vi "Emballage_BDD_lecutreCommandeNonTerminé.vi"(8 "entrée d'erreur (pas d'erreur)":errorcluster) -> (0 "sortie d'erreur":errorcluster, 2 "Cmd_nonFini":string[](array[string]), 3 "Liste des champs à lire 2":string[][](array[string]))   [LabVIEW 2020]
uses:
  Modules/FS/60_FS_Controles/60_FS_SetGet.ctl
  <vilib>/addons/database/Connection.llb/DB Tools Open Connec (Path).vi
  <vilib>/addons/database/Connection.llb/Conn Execute.vi
  <vilib>/addons/database/Recordset.llb/Rec Fetch Recordset Data (R).vi
  <vilib>/addons/database/Recordset.llb/Rec Destroy - Connection.vi
  <vilib>/addons/database/NI_Database_API.lvlib
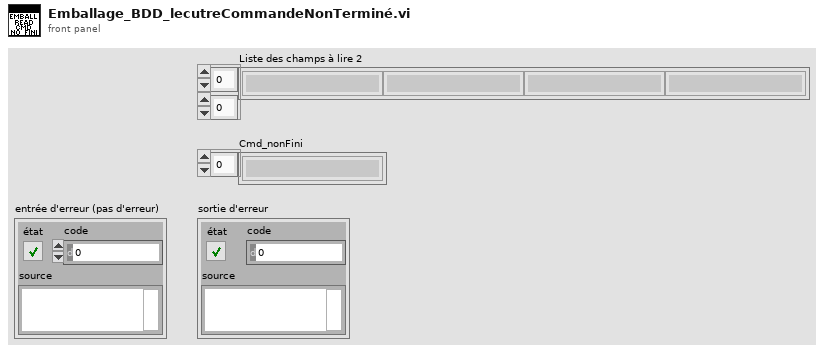
[diagram p1: front panel]
types:
  T1 = typedef "60_FS_SetGet.ctl" = enum16{"set", "get"}
  T2 = typedef "Emballage_BDD_param_Produit.ctl" = cluster{"No_Valve_FAS":string, "suffixe":string, "designation":string, "indice_produit":string, "code_barre_fixe":string, "affiche_code_barre_client":string, "affiche_no_client":string, "Nb_vlve_par_carton":u16, "melange_des_lots_possible":string, "id_article":string, "Indice_Rev":string, "Famille":string, "date":string, "code_barre_fixe_Fin":string, "Longeur_No_Serie":string}
  T3 = typedef "60_FS_CLT_Chemins.ctl" = cluster{"Racine_local":path, "Racine_reseau":path, "Racine_Support_Application":path, "Fichier_Journalisation":path, "Connexion_BDD_VSX":path, "Connexion_BDD_PLZ":path}
  T4 = typedef "NI_Database_API.lvlib/Conn ObjectReference.ctl" = refnum<k1>
  T5 = typedef "NI_Database_API.lvlib/Rec ObjectReference.ctl" = refnum<k1>
  T6 = typedef "DATA commande.ctl" = cluster{"n°article FAS":string, "n° cmde FAS":string, "quantité cmde":string, "ID LIG cmde":string, "n° cmde client":string, "nom client":string, "n° article client":string, "indice revision client":string, "société de facturation":string, "langue a utiliser":string}
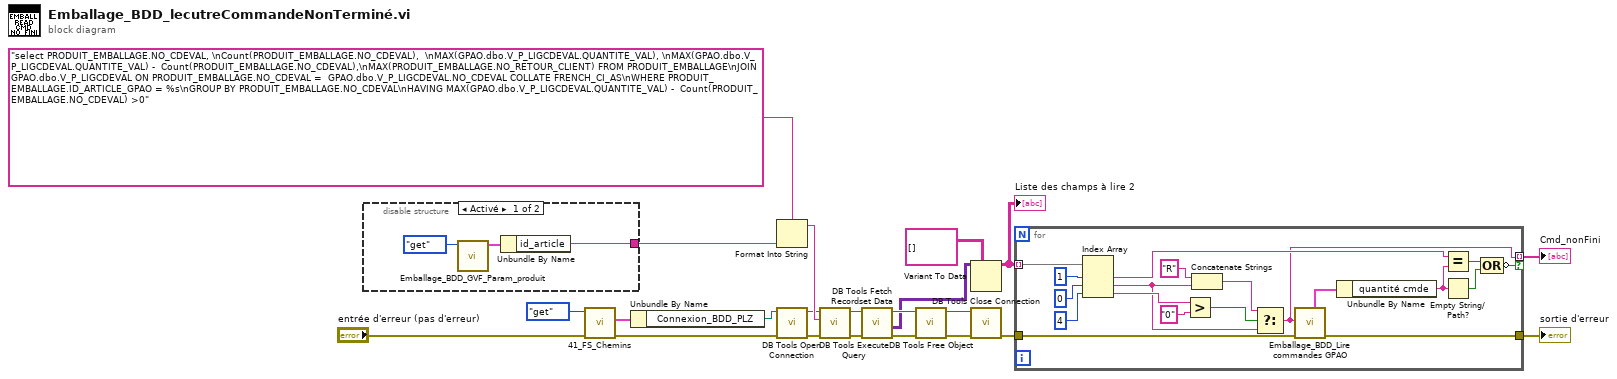
[diagram p0: block diagram]
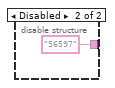
[diagram p2: hidden frame]
diagram:
  n1 = disable-structure shown="Activé" {
    disable-tunnel: [w25 "56597" ("id_article")] -> w16
    frame Enabled {
      n2 = call "Emballage_BDD_GVF_Param_produit.vi"("Énum"=enum16{"set", "get"}."get") -> ("CLS_param_produit"=w23:T2)  [unwired: 7 in, 3 out]
      n3 = Unbundle By Name(w23) -> ("id_article"=w25:string)
    }
    frame Disabled {
    }
  }
  n4 = call "41_FS_Chemins.vi"("error in (no error)"="entrée d'erreur (pas d'erreur)", "SetGet"=60_FS_SetGet."get") -> ("error out"=w4:errorcluster, "CLT_Chemins_out"=w1:T3)  [unwired: 8 in]
  n5 = Unbundle By Name(w1) -> ("Connexion_BDD_PLZ"=w7:path)
  n6 = Format Into String(format string="select PRODUIT_EMBALLAGE.NO_CDEVAL, \nCount(PRODUIT_EMBALLAGE.NO_CDEVAL),  \nMAX(GPAO.dbo.V_P_LIGCDEVAL.QUANTITE_VAL), \nMAX(GPAO.dbo.V_P_LIGCDEVAL.QUANTITE_VAL) -  Count(PRODUIT_EMBALLAGE.NO_CDEVAL),\nMAX(PRODUIT_EMBALLAGE.NO_RETOUR_CLIENT) FROM PRODUIT_EMBALLAGE\nJOIN GPAO.dbo.V_P_LIGCDEVAL ON PRODUIT_EMBALLAGE.NO_CDEVAL =  GPAO.dbo.V_P_LIGCDEVAL.NO_CDEVAL COLLATE FRENCH_CI_AS\nWHERE PRODUIT_EMBALLAGE.ID_ARTICLE_GPAO = %s\nGROUP BY PRODUIT_EMBALLAGE.NO_CDEVAL\nHAVING MAX(GPAO.dbo.V_P_LIGCDEVAL.QUANTITE_VAL) -  Count(PRODUIT_EMBALLAGE.NO_CDEVAL) >0" ("SQL query"), w16) -> (resulting string=w14:string)  [unwired: 2 in, 1 out]
  n7 = call-poly <vilib>:"DB Tools Open Connection.vi"("error in (no error)"=w4, "connection information"=w7) -> ("error out"=w5:errorcluster, "connection reference"=w6:T4)  [unwired: 6 in]
  n8 = call-poly <vilib>:"DB Tools Execute Query.vi"("error in (no error)"=w5, "SQL query"=w14, "connection reference"=w6) -> ("error out"=w8:errorcluster, "recordset reference"=w9:T5)  [unwired: 5 in]
  n9 = call-poly <vilib>:"DB Tools Fetch Recordset Data.vi"("error in (no error)"=w8, "recordset reference"=w9) -> ("error out"=w19:errorcluster, "recordset data"=w11:variant[][], "recordset reference out"=w21:T5)  [unwired: 3 in]
  n10 = call-poly <vilib>:"DB Tools Free Object.vi"("error in (no error)"=w19, "recordset reference"=w21) -> ("error out"=w18:errorcluster, "connection reference"=w22:T4)  [unwired: 8 in]
  n11 = Variant To Data(type=string[][] [] ("Liste des champs à lire 2"), Variant=w11) -> (data=w17:string[][])  [unwired: 1 in, 1 out]
  "Liste des champs à lire 2" <- w17
  n12 = call <vilib>:"DB Tools Close Connection.vi"("error in (no error)"=w18, "connection reference"=w22) -> ("error out"=w20:errorcluster)  [unwired: 5 in]
  n13 = for {
    tunnel: [w27] -> w13 mode=indexing if=w41
    tunnel: w20 -> [w40]
    tunnel: [w39] -> w12
    tunnel: w17 -> [w38] mode=indexing
    n14 = Index Array(array=w38, index #1=1 ("indice"), index #2=0 ("indice"), index #3=4 ("index")) -> (element #1=w35:string, element #2=w28:string, element #3=w33:string)
    n15 = Greater?(x=w33, y="0") -> (0:w31:bool)
    n16 = Concatenate Strings("R" ("string"), w28) -> (w30:string)
    n17 = Select(t=w30, s=w31, f=w28) -> (s? t:f=w27:string)
    n18 = call "Emballage_BDD_Lire  commandes GPAO.vi"("error in"=w40, "Numéro commande"=w27) -> ("error out"=w39:errorcluster, "DATA cmde"=w45:T6)  [unwired: 4 in, 4 out]
    n19 = Unbundle By Name(w45) -> ("quantité cmde"=w43:string)
    n20 = Equal?(x=w35, y=w43) -> (x = y?=w44:bool)
    n21 = Empty String/Path?(string/path=w43) -> (empty?=w42:bool)
    n22 = Compound Arithmetic op=OR ("Opérateur arithmétique")(w44, w42) -> (invert w41:bool)
  }
  "Cmd_nonFini" <- w13
  "sortie d'erreur" <- w12
